vi "QMH_Daq.vi"(8 "Error In":errorcluster, 10 "DaQ Queue In":refnum<queue>, 11 "QMH Queue":refnum<queue>) -> (2 "DaQ Queue Out":refnum<queue>, 3 "QMH Queue Out":refnum<queue>)   [LabVIEW 2021, in "Main.lvlib" / "Main_Programs_SubVIs.lvlib"]
doc: "This VI is the QMH loop for the DaQ operation."
uses:
  Main_Programs_SubVIs.lvlib
  Tipski Definicii/QMH_Daq_States.ctl
  Tipski Definicii/error_handl.ctl
  Polymorphic/DeQ_DaQ_QMH.vi
  Polymorphic/Enq_DaQ_QMH.vi
  Polymorphic/DaQ_Signal_Deq.vi
  Main.lvlib
  Polymorphic/Queues.lvlib
panel:
  # "Output"
  # "Input"
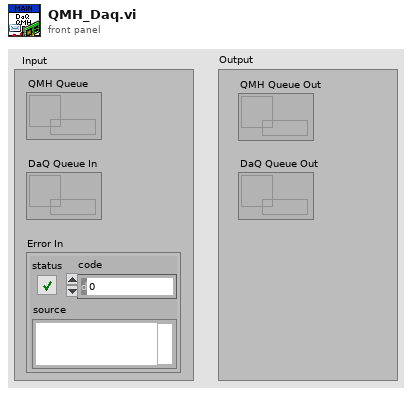
[diagram p1: front panel]
types:
  T1 = typedef "error_handl.ctl" = enum16{"Init", "Insert Error 1", "Insert Error 2", "Insert Error 3", "Insert Error 4", "Handle Erros"}
  T2 = typedef "QMH_Daq_States.ctl" = enum16{"Idle", "Start DaQ", "DaQ", "Generate Message", "Stop DaQ", "End"}
  T3 = enum16{"Init", "Init DaQ", "Start", "Output", "Stop", "Delete", "V/A ?"}
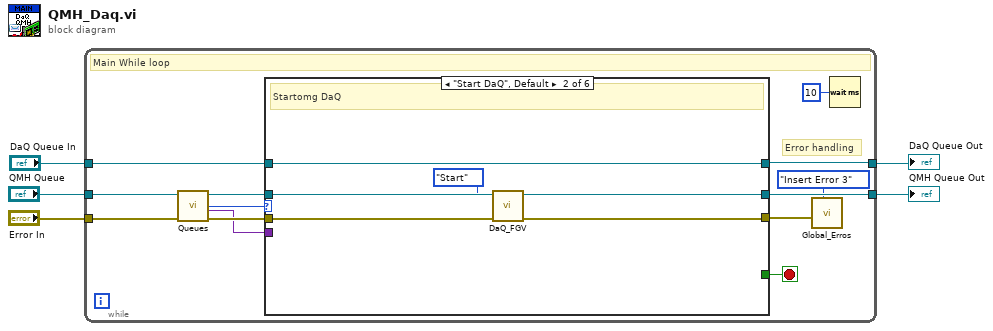
[diagram p0: block diagram]
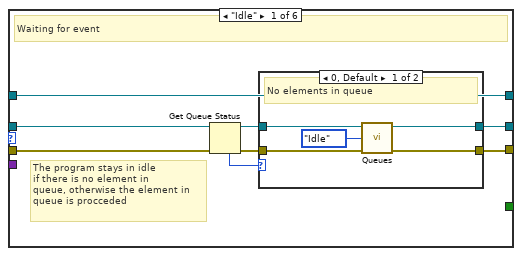
[diagram p2: hidden frame]
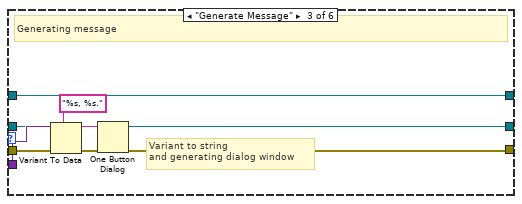
[diagram p4: hidden frame]
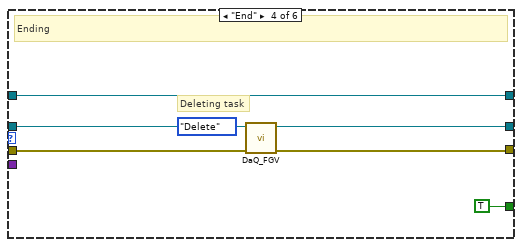
[diagram p5: hidden frame]
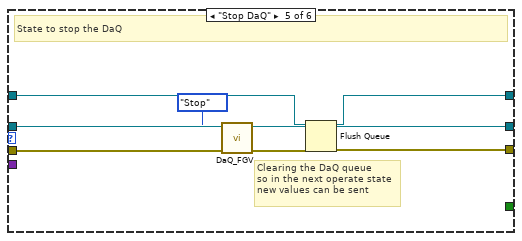
[diagram p6: hidden frame]
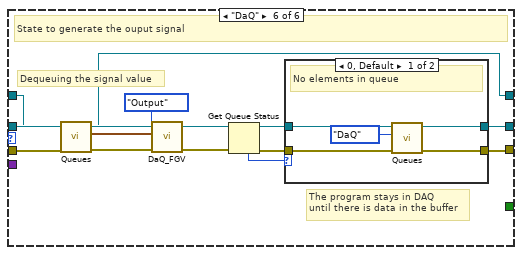
[diagram p7: hidden frame]
diagram:
  n1 = while {
    tunnel: "QMH Queue" -> [w11]
    tunnel: "Error In" -> [w16]
    tunnel: [w18] -> w3
    tunnel: "DaQ Queue In" -> [w10]
    tunnel: [w6] -> w1
    stop <- w17 stop-if-true
    # "Error handling"
    # "Main While loop"
    n2 = call-poly "Queues.vi"("Error In"=w16, "Queue In"=w11) -> ("Error Out"=w14:errorcluster, "Message"=w13:variant, "Instruction"=w12:T2, "Queue Out"=w15:refnum<queue>)  [unwired: 6 in]
    n3 = case shown="\"Start DaQ\", Default" w12 {
      tunnel: w13 -> [_ _ w45 _ _ _]
      tunnel: w14 -> [w25 w37 w44 w49 w57 w65]
      tunnel: w15 -> [w26 w38 w41 w51 w58 w71]
      tunnel: [w22 w38 w41 w51 w58 w67] -> w18
      tunnel: [w20 w36 w40 w48 w55 w66] -> w8
      tunnel: [_ _ _ TRUE _ _] -> w17
      tunnel: w10 -> [w19 w34 w39 w46 w54 w64]
      tunnel: [w19 w34 w39 w46 w53 w59] -> w6
      frame "Idle" {
        # "The program stays in idle\nif there is no element in \nqueue, otherwise the element in \nqueue is procceded"
        # "Waiting for event"
        n4 = Get Queue Status(queue=w26, error in (no error)=w25) -> (queue out=w23:refnum<queue>, error out=w21:errorcluster, # elements in queue=w24:i32)  [unwired: 1 in, 5 out]
        n5 = case shown="0, Default" w24 {
          tunnel: [w29 w33] -> w22
          tunnel: w23 -> [w30 w33]
          tunnel: w21 -> [w31 w32]
          tunnel: [w28 w32] -> w20
          frame 0, Default {
            # "No elements in queue"
            n6 = call-poly "Queues.vi"("Error In"=w31, "Instruction"=QMH_Daq_States."Idle", "Queue In"=w30) -> ("Error Out"=w28:errorcluster, "Queue Out"=w29:refnum<queue>)  [unwired: 7 in]
          }
          frame 1.. {
            # "One or more elements in queue"
          }
        }
      }
      frame "Start DaQ", Default {
        # "Startomg DaQ"
        n7 = call "DaQ_FGV.vi"("Error In"=w37, "Action"=T3."Start") -> ("Error Out"=w36:errorcluster)  [unwired: 9 in]
      }
      frame "Generate Message" {
        # "Variant to string\nand generating dialog window"
        # "Generating message"
        n8 = Variant To Data(error in=w44, type="%s, %s.", Variant=w45) -> (data=w42:string, error out=w40:errorcluster)
        n9 = One Button Dialog(message=w42) -> ()  [unwired: 1 in, 1 out]
      }
      frame "End" {
        # "Deleting task"
        # "Ending"
        n10 = call "DaQ_FGV.vi"("Error In"=w49, "Action"=T3."Delete") -> ("Error Out"=w48:errorcluster)  [unwired: 9 in]
      }
      frame "Stop DaQ" {
        # "Clearing the DaQ queue \nso in the next operate state\nnew values can be sent"
        # "State to stop the DaQ"
        n11 = call "DaQ_FGV.vi"("Error In"=w57, "Action"=T3."Stop") -> ("Error Out"=w52:errorcluster)  [unwired: 9 in]
        n12 = Flush Queue(queue=w54, error in (no error)=w52) -> (queue out=w53:refnum<queue>, error out=w55:errorcluster)  [unwired: 1 out]
      }
      frame "DaQ" {
        # "Dequeuing the signal value"
        # "The program stays in DAQ\nuntil there is data in the buffer"
        # "State to generate the ouput signal"
        n13 = call-poly "Queues.vi"("Error In"=w65, "Queue In"=w64) -> ("Error Out"=w63:errorcluster, "Signal"=w60:waveform(dbl), "Queue Out"=w59:refnum<queue>)  [unwired: 7 in]
        n14 = call "DaQ_FGV.vi"("Error In"=w63, "Output Signal"=w60, "Action"=T3."Output") -> ("Error Out"=w62:errorcluster)  [unwired: 8 in]
        n15 = Get Queue Status(queue=w71, error in (no error)=w62) -> (queue out=w69:refnum<queue>, error out=w68:errorcluster, # elements in queue=w70:i32)  [unwired: 1 in, 5 out]
        n16 = case shown="0, Default" w70 {
          tunnel: w69 -> [w76 w77]
          tunnel: w68 -> [w75 w78]
          tunnel: [w73 w77] -> w67
          tunnel: [w72 w78] -> w66
          frame 0, Default {
            # "No elements in queue"
            n17 = call-poly "Queues.vi"("Error In"=w75, "Instruction"=QMH_Daq_States."DaQ", "Queue In"=w76) -> ("Error Out"=w72:errorcluster, "Queue Out"=w73:refnum<queue>)  [unwired: 7 in]
          }
          frame 1.. {
            # "One or more elements in queue"
          }
        }
      }
    }
    n18 = call "Global_Erros.vi"("Action"=error_handl."Insert Error 3", "Error Loop 3"=w8) -> ()  [unwired: 9 in, 1 out]
    n19 = Wait (ms)(milliseconds to wait=u32 10) -> ()  [unwired: 1 out]
  }
  "QMH Queue Out" <- w3
  "DaQ Queue Out" <- w1
